vi "(De)Activate Cell.vi"(8 "error in (no error)":errorcluster, 10 "Active":bool=TRUE, 11 "Schedule Cell in":refnum<class "Schedule Cell.lvclass">) -> (0 "error out":errorcluster, 3 "Schedule Cell out":refnum<class "Schedule Cell.lvclass">)   [LabVIEW 2020, in "TALOS.lvlib" / "Run Utilities.lvlib" / "Schedule Cell.lvclass"]
doc: "Set activate flag to true of false"
uses:
  Schedule Cell.lvclass
  Schedule Cell.lvclass/Schedule Cell.ctl
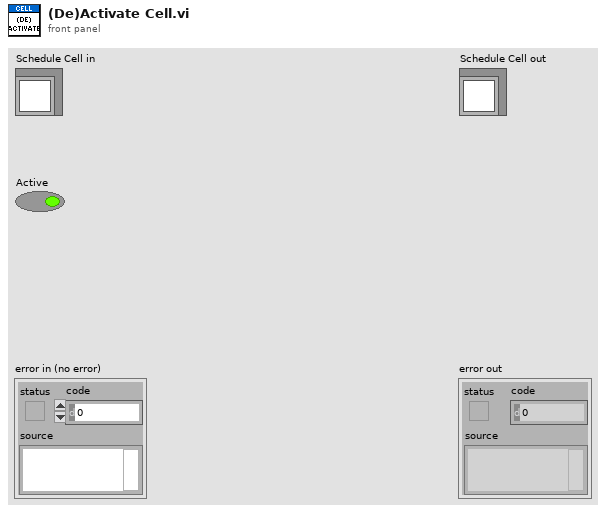
[diagram p1: front panel]
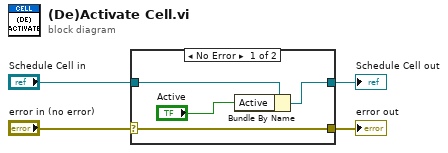
[diagram p0: block diagram]
diagram:
  n1 = case shown="No Error" "error in (no error)" {
    selector: "error in (no error)" -> [w8 w10]
    tunnel: [w8 w10] -> w3
    tunnel: [w6 w9] -> w1
    tunnel: "Schedule Cell in" -> [w7 w9]
    frame No Error {
      n2 = Bundle By Name(cluster=w7, "Active"="Active") -> (w6:refnum<class "Schedule Cell.lvclass">)
    }
    frame Error {
    }
  }
  "error out" <- w3
  "Schedule Cell out" <- w1
